vi "n3_bis_betas.vi"(4 "Time":dbl[](array[numeric]), 5 "Tamaño Sn":i32[](array[numeric]), 6 "Analysis":u8, 8 "m":dbl, 9 "P":dbl, 10 "Segmentation A":dbl[](array[numeric]), 11 "Segmentation B":dbl[](array[numeric])) -> (0 "bB":dbl, 1 "X2_tau":dbl[][](array[numeric]), 2 "X2_i":dbl[][](array[numeric]), 3 "bA":dbl)   [LabVIEW 2015]
uses:
  <vilib>/Analysis/baseanly.llb/Mean (DBL).vi
  <vilib>/Analysis/NI_AALBase.lvlib
  <vilib>/Analysis/NI_AALPro.lvlib
panel:
  out "bB_anterior":dbl
  out "bA_anterior":dbl
  out "amplitude 2":dbl
  out "offset 2":dbl
  out "offset":dbl
  out "time":dbl[](array[numeric])
  out "amplitude":dbl
  out "output array 4":dbl[](array[numeric])
  out "Canelos":dbl[](array[numeric])
  out "MA 3":dbl
  out "MB 2":dbl
  out "MA 2":dbl
  out "output array 2":dbl[](array[numeric])
  out "MB":dbl
  out "MA":dbl
  out "output array":dbl[](array[numeric])
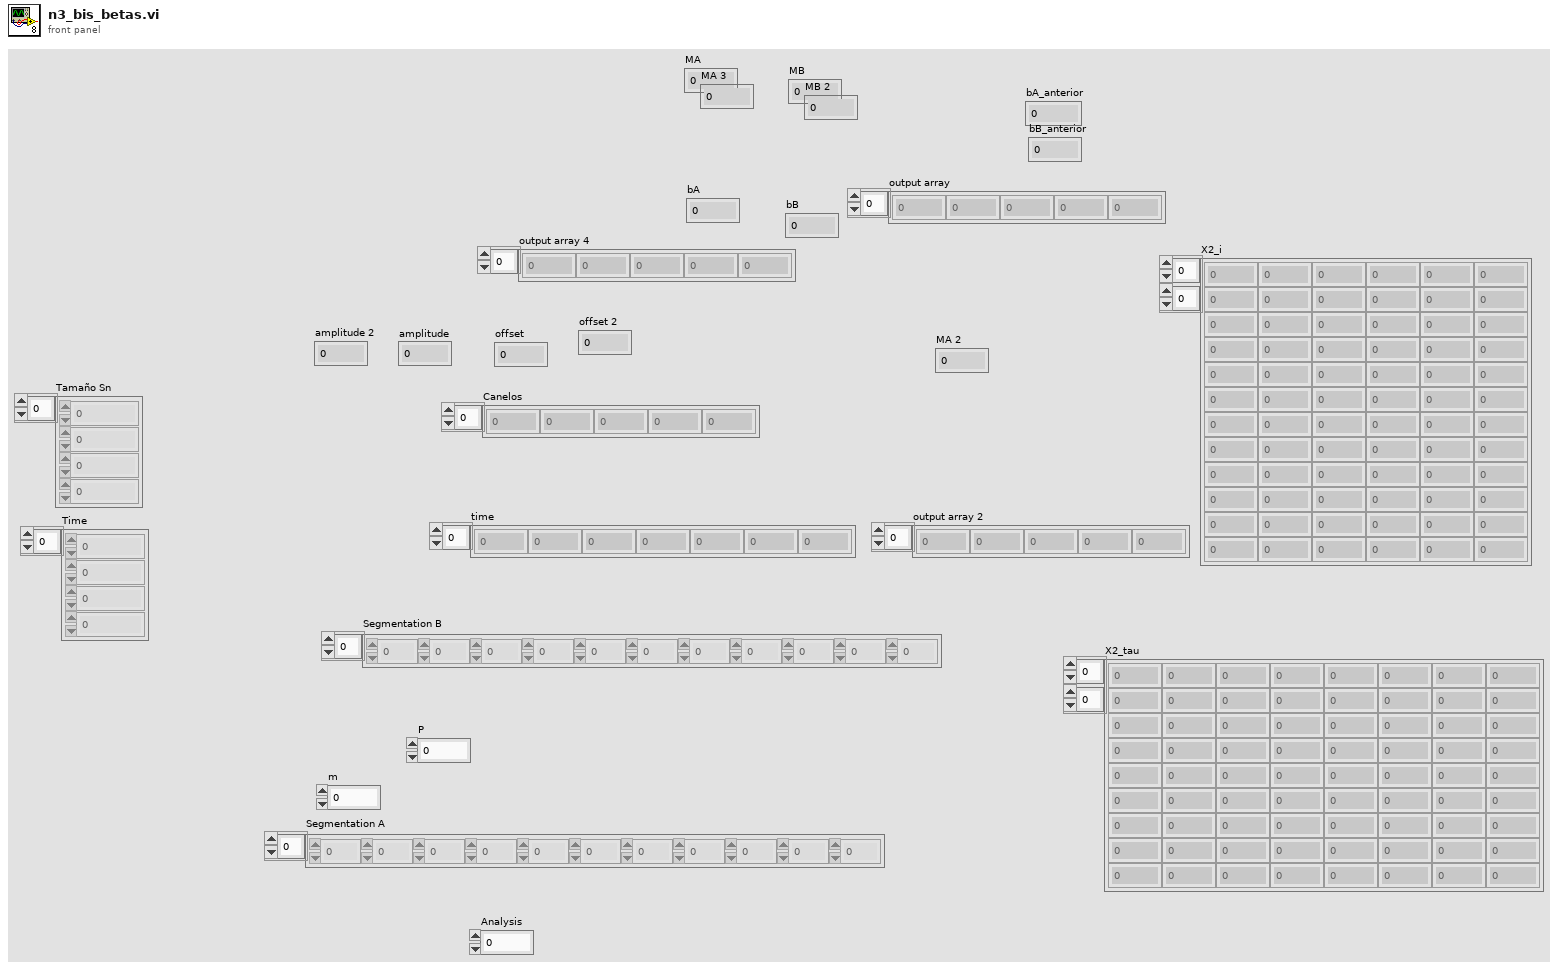
[diagram p1: front panel]
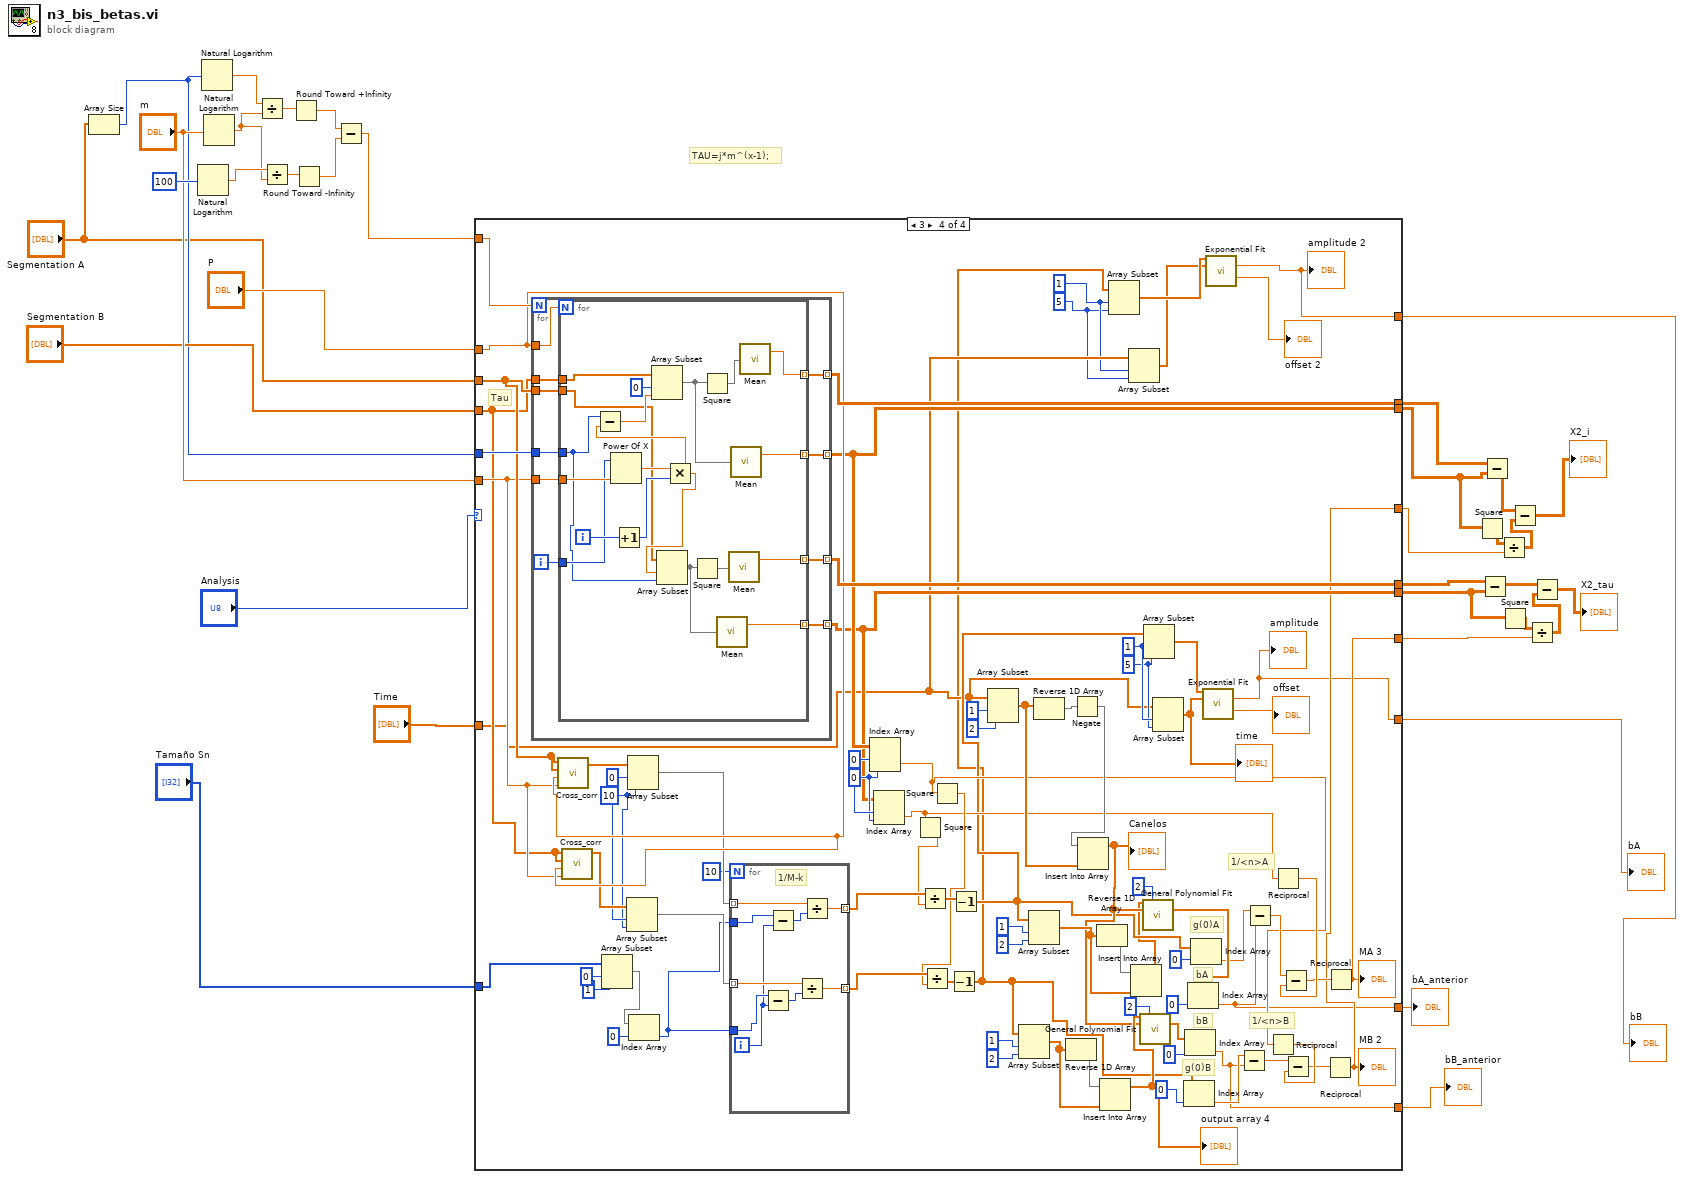
[diagram p0: block diagram]
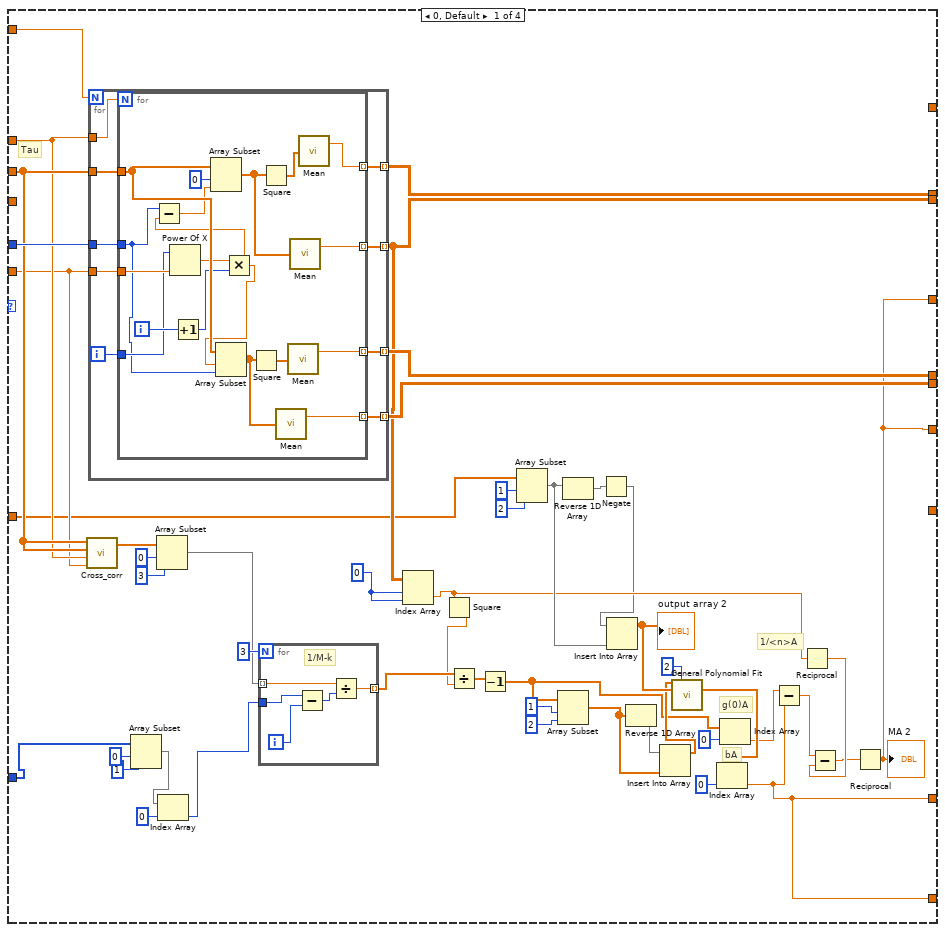
[diagram p2: hidden frame]
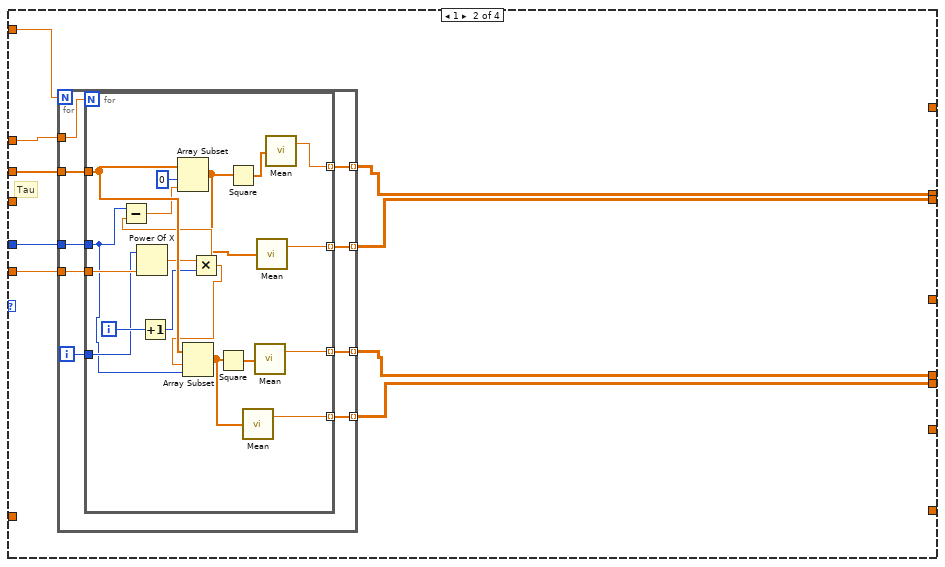
[diagram p3: hidden frame]
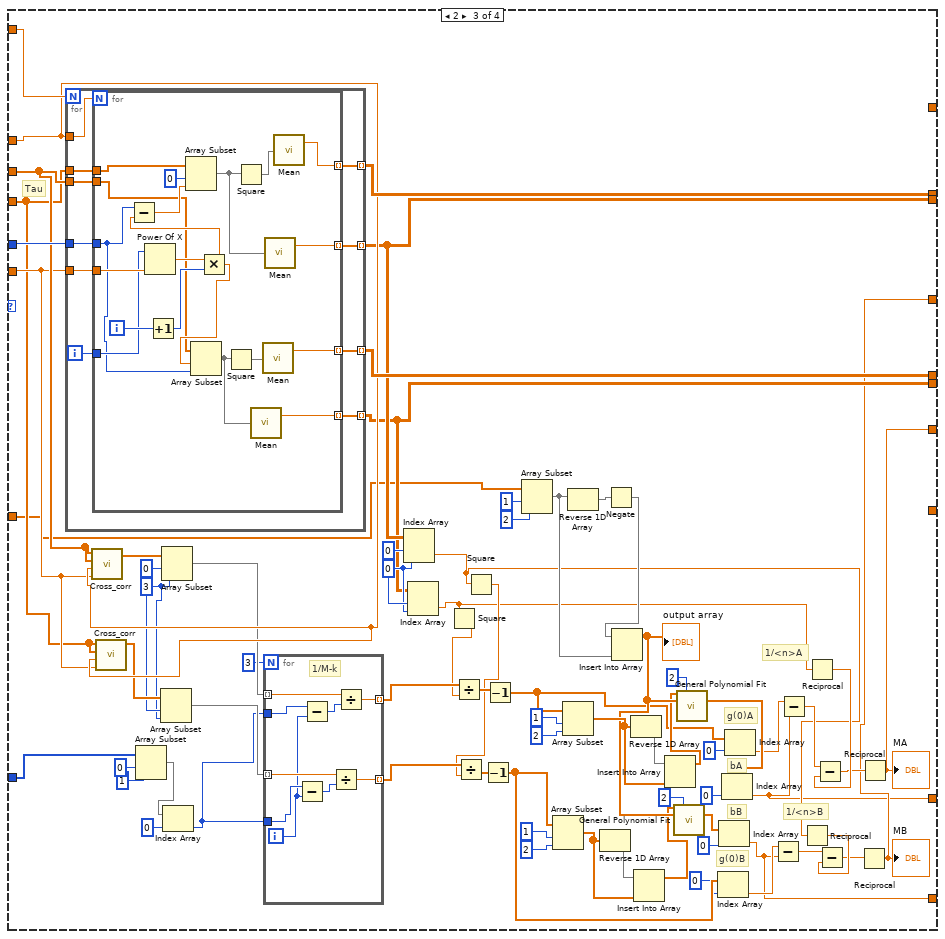
[diagram p4: hidden frame]
diagram:
  # "TAU=j*m^(x-1);"
  n1 = Array Size(array="Segmentation A") -> (size(s)=w20:i32)
  n2 = Natural Logarithm(1:100) -> (0:w32:dbl)
  n3 = Natural Logarithm(1:w20) -> (0:w35:dbl)
  n4 = Natural Logarithm(1:"m") -> (0:w31:dbl)
  n5 = Divide(x=w35, y=w31) -> (x/y=w34:dbl)
  n6 = Divide(x=w32, y=w31) -> (x/y=w29:dbl)
  n7 = Round Toward +Infinity(x=w34) -> (ceil(x): smallest int >= x=w30:dbl)
  n8 = Round Toward -Infinity(1:w29) -> (0:w28:dbl)
  n9 = Subtract(x=w30, y=w28) -> (x-y=w27:dbl)
  n10 = case shown="3" "Analysis" {
    tunnel: "Segmentation A" -> [w47 w124 w219 w341]
    tunnel: w20 -> [w79 w123 w222 w344]
    tunnel: w27 -> [w80 w122 w223 w345]
    tunnel: "m" -> [w45 w121 w217 w339]
    tunnel: "P" -> [w46 w120 w218 w340]
    tunnel: [w83 w119 w221 w343] -> w22
    tunnel: [w42 w118 w204 w326] -> w16
    tunnel: [w82 w117 w220 w342] -> w21
    tunnel: [w81 w116 w179 w304] -> w17
    tunnel: "Segmentation B" -> [_ _ w158 w285]
    tunnel: "Tamaño Sn" -> [w48 _ w210 w332]
    tunnel: [w41 _ w157 w284] -> w14
    tunnel: [w41 _ w156 w283] -> w9
    tunnel: "Time" -> [w37 _ w154 w270]
    tunnel: [w36 _ w153 w281] -> w2
    tunnel: [w36 _ w152 w280] -> w1
    tunnel: [_ _ _ w265] -> w4
    tunnel: [_ _ _ w264] -> w3
    frame 0, Default {
      w43 = 0 ("index (col)")
      # "1/<n>A"
      # "bA"
      # "g(0)A"
      # "Tau"
      n11 = call "Cross_corr.vi"("m"=w45, "P"=w46, "input B"=w47, "input A"=w47) -> ("Acc"=w78:dbl[])  [unwired: 5 in, 2 out]
      n12 = for {
        N: w80 -> [_]
        tunnel: w46 -> [w97]
        tunnel: w47 -> [w96]
        tunnel: w79 -> [w95]
        tunnel: w45 -> [w94]
        tunnel: [w93] -> w83 mode=indexing
        tunnel: [w92] -> w42 mode=indexing
        tunnel: [w90] -> w82 mode=indexing
        tunnel: [w89] -> w81 mode=indexing
        i -> [w91]
        n13 = for {
          N: w97 -> [_]
          tunnel: w96 -> [w112]
          tunnel: w95 -> [w104]
          tunnel: w94 -> [w115]
          tunnel: w91 -> [w106]
          tunnel: [w114] -> w93 mode=indexing
          tunnel: [w113] -> w92 mode=indexing
          tunnel: [w110] -> w90 mode=indexing
          tunnel: [w109] -> w89 mode=indexing
          i -> [w108]
          n14 = Power Of X(1:w115, 2:w106) -> (0:w98:dbl)
          n15 = Increment(x=w108) -> (x+1=w107:i32)
          n16 = Multiply(x=w98, y=w107) -> (x*y=w105:dbl)
          n17 = Subtract(x=w104, y=w105) -> (x-y=w102:dbl)
          n18 = Array Subset(array=w112, index=0, length=w102) -> (w103:dbl[])
          n19 = Array Subset(array=w112, index=w105, length=w104) -> (w99:dbl[])
          n20 = Square(x=w99) -> (x^2=w111:dbl[])
          n21 = Square(x=w103) -> (x^2=w100:dbl[])
          n22 = call-poly <vilib>:"Mean.vi"("X"=w99) -> ("mean"=w109:dbl)  [unwired: 1 out]
          n23 = call-poly <vilib>:"Mean.vi"("X"=w111) -> ("mean"=w110:dbl)  [unwired: 1 out]
          n24 = call-poly <vilib>:"Mean.vi"("X"=w103) -> ("mean"=w113:dbl)  [unwired: 1 out]
          n25 = call-poly <vilib>:"Mean.vi"("X"=w100) -> ("mean"=w114:dbl)  [unwired: 1 out]
        }
      }
      n26 = Array Subset(array=w48, index=0, length=1) -> (w73:i32[])
      n27 = Array Subset(array=w78, index=0, length=3) -> (w39:dbl[])
      n28 = Index Array(array=w73, index=0) -> (element=w44:i32)
      n29 = for {
        N: 3 -> [_]
        tunnel: w39 -> [w87] mode=indexing
        tunnel: w44 -> [w86]
        tunnel: [w84] -> w71 mode=indexing
        i -> [w85]
        # "1/M-k"
        n30 = Subtract(x=w86, y=w85) -> (x-y=w88:i32)
        n31 = Divide(x=w87, y=w88) -> (x/y=w84:dbl)
      }
      n32 = Index Array(array=w42, index (row)=w43, index (col)=w43) -> (element=w52:dbl)
      n33 = Square(x=w52) -> (x^2=w58:dbl)
      n34 = Divide(x=w71, y=w58) -> (x/y=w70:dbl[])
      n35 = Decrement(x=w70) -> (x-1=w57:dbl[])
      n36 = Array Subset(array=w37, index=1, length=2) -> (w62:dbl[])
      n37 = Array Subset(array=w57, index=1, length=2) -> (w61:dbl[])
      n38 = Reverse 1D Array(array=w62) -> (reversed array=w67:dbl[])
      n39 = Negate(x=w67) -> (-x=w38:dbl[])
      n40 = Insert Into Array(array=w38, new element=w62) -> (w60:dbl[])  [unwired: 1 in]
      "output array 2" <- w60
      n41 = Reverse 1D Array(array=w61) -> (reversed array=w63:dbl[])
      n42 = Insert Into Array(array=w63, new element=w61) -> (w59:dbl[])  [unwired: 1 in]
      n43 = call <vilib>:"General Polynomial Fit.vi"("Y"=w59, "polynomial order"=2, "X"=w60) -> ("Polynomial Coefficients"=w55:dbl[])  [unwired: 9 in, 3 out]
      n44 = Index Array(array=w55, index=0) -> (element=w36:dbl)
      n45 = Index Array(array=w57, index=0) -> (element=w53:dbl)
      n46 = Subtract(x=w53, y=w36) -> (x-y=w51:dbl)
      n47 = Reciprocal(x=w52) -> (1/x=w50:dbl)
      n48 = Subtract(x=w51, y=w50) -> (x-y=w49:dbl)
      n49 = Reciprocal(x=w49) -> (1/x=w41:dbl)
      "MA 2" <- w41
    }
    frame 1 {
      # "Tau"
      n50 = for {
        N: w122 -> [_]
        tunnel: w120 -> [w133]
        tunnel: w124 -> [w132]
        tunnel: w123 -> [w131]
        tunnel: w121 -> [w130]
        tunnel: [w129] -> w119 mode=indexing
        tunnel: [w128] -> w118 mode=indexing
        tunnel: [w126] -> w117 mode=indexing
        tunnel: [w125] -> w116 mode=indexing
        i -> [w127]
        n51 = for {
          N: w133 -> [_]
          tunnel: w132 -> [w148]
          tunnel: w131 -> [w138]
          tunnel: w130 -> [w151]
          tunnel: w127 -> [w141]
          tunnel: [w150] -> w129 mode=indexing
          tunnel: [w149] -> w128 mode=indexing
          tunnel: [w146] -> w126 mode=indexing
          tunnel: [w144] -> w125 mode=indexing
          i -> [w143]
          n52 = Power Of X(1:w151, 2:w141) -> (0:w140:dbl)
          n53 = Increment(x=w143) -> (x+1=w142:i32)
          n54 = Multiply(x=w140, y=w142) -> (x*y=w139:dbl)
          n55 = Subtract(x=w138, y=w139) -> (x-y=w136:dbl)
          n56 = Array Subset(array=w148, index=0, length=w136) -> (w137:dbl[])
          n57 = Array Subset(array=w148, index=w139, length=w138) -> (w145:dbl[])
          n58 = Square(x=w145) -> (x^2=w147:dbl[])
          n59 = Square(x=w137) -> (x^2=w134:dbl[])
          n60 = call-poly <vilib>:"Mean.vi"("X"=w145) -> ("mean"=w144:dbl)  [unwired: 1 out]
          n61 = call-poly <vilib>:"Mean.vi"("X"=w147) -> ("mean"=w146:dbl)  [unwired: 1 out]
          n62 = call-poly <vilib>:"Mean.vi"("X"=w137) -> ("mean"=w149:dbl)  [unwired: 1 out]
          n63 = call-poly <vilib>:"Mean.vi"("X"=w134) -> ("mean"=w150:dbl)  [unwired: 1 out]
        }
      }
    }
    frame 2 {
      w202 = 0 ("index (col)")
      w203 = 0 ("index (row)")
      w155 = 3 ("length")
      w214 = 0 ("index")
      # "1/<n>B"
      # "1/<n>A"
      # "bB"
      # "bA"
      # "g(0)B"
      # "g(0)A"
      # "Tau"
      n64 = for {
        N: w223 -> [_]
        tunnel: w218 -> [w242]
        tunnel: w158 -> [w241]
        tunnel: w222 -> [w240]
        tunnel: w217 -> [w239]
        tunnel: [w238] -> w221 mode=indexing
        tunnel: [w237] -> w204 mode=indexing
        tunnel: [w235] -> w220 mode=indexing
        tunnel: [w234] -> w179 mode=indexing
        tunnel: w219 -> [w233]
        i -> [w236]
        n65 = for {
          N: w242 -> [_]
          tunnel: w241 -> [w244]
          tunnel: w240 -> [w249]
          tunnel: w239 -> [w261]
          tunnel: w236 -> [w252]
          tunnel: [w260] -> w238 mode=indexing
          tunnel: [w259] -> w237 mode=indexing
          tunnel: [w257] -> w235 mode=indexing
          tunnel: [w255] -> w234 mode=indexing
          tunnel: w233 -> [w243]
          i -> [w254]
          n66 = Power Of X(1:w261, 2:w252) -> (0:w251:dbl)
          n67 = Increment(x=w254) -> (x+1=w253:i32)
          n68 = Multiply(x=w251, y=w253) -> (x*y=w250:dbl)
          n69 = Subtract(x=w249, y=w250) -> (x-y=w247:dbl)
          n70 = Array Subset(array=w244, index=0, length=w247) -> (w248:dbl[])
          n71 = Array Subset(array=w243, index=w250, length=w249) -> (w256:dbl[])
          n72 = Square(x=w256) -> (x^2=w258:dbl[])
          n73 = Square(x=w248) -> (x^2=w245:dbl[])
          n74 = call-poly <vilib>:"Mean.vi"("X"=w256) -> ("mean"=w255:dbl)  [unwired: 1 out]
          n75 = call-poly <vilib>:"Mean.vi"("X"=w258) -> ("mean"=w257:dbl)  [unwired: 1 out]
          n76 = call-poly <vilib>:"Mean.vi"("X"=w248) -> ("mean"=w259:dbl)  [unwired: 1 out]
          n77 = call-poly <vilib>:"Mean.vi"("X"=w245) -> ("mean"=w260:dbl)  [unwired: 1 out]
        }
      }
      n78 = call "Cross_corr.vi"("m"=w217, "P"=w218, "input B"=w219, "input A"=w219) -> ("Acc"=w216:dbl[])  [unwired: 5 in, 2 out]
      n79 = call "Cross_corr.vi"("m"=w217, "P"=w218, "input B"=w158, "input A"=w158) -> ("Acc"=w215:dbl[])  [unwired: 5 in, 2 out]
      n80 = Array Subset(array=w210, index=0, length=1) -> (w207:i32[])
      n81 = Array Subset(array=w215, index=w214, length=w155) -> (w212:dbl[])
      n82 = Array Subset(array=w216, index=w214, length=w155) -> (w213:dbl[])
      n83 = Index Array(array=w207, index=0) -> (element=w205:i32)
      n84 = for {
        N: 3 -> [_]
        tunnel: [w232] -> w200 mode=indexing
        tunnel: w212 -> [w231] mode=indexing
        tunnel: w205 -> [w229]
        tunnel: w213 -> [w227] mode=indexing
        tunnel: w205 -> [w226]
        tunnel: [w224] -> w201 mode=indexing
        i -> [w225]
        # "1/M-k"
        n85 = Subtract(x=w229, y=w225) -> (x-y=w230:i32)
        n86 = Subtract(x=w226, y=w225) -> (x-y=w228:i32)
        n87 = Divide(x=w231, y=w230) -> (x/y=w232:dbl)
        n88 = Divide(x=w227, y=w228) -> (x/y=w224:dbl)
      }
      n89 = Index Array(array=w204, index (row)=w203, index (col)=w202) -> (element=w160:dbl)
      n90 = Index Array(array=w179, index (row)=w203, index (col)=w202) -> (element=w167:dbl)
      n91 = Square(x=w167) -> (x^2=w177:dbl)
      n92 = Divide(x=w201, y=w177) -> (x/y=w199:dbl[])
      n93 = Square(x=w160) -> (x^2=w178:dbl)
      n94 = Divide(x=w200, y=w178) -> (x/y=w198:dbl[])
      n95 = Decrement(x=w198) -> (x-1=w174:dbl[])
      n96 = Decrement(x=w199) -> (x-1=w176:dbl[])
      n97 = Array Subset(array=w154, index=1, length=2) -> (w189:dbl[])
      n98 = Array Subset(array=w174, index=1, length=2) -> (w183:dbl[])
      n99 = Array Subset(array=w176, index=1, length=2) -> (w188:dbl[])
      n100 = Reverse 1D Array(array=w189) -> (reversed array=w195:dbl[])
      n101 = Reverse 1D Array(array=w183) -> (reversed array=w184:dbl[])
      n102 = Negate(x=w195) -> (-x=w194:dbl[])
      n103 = Insert Into Array(array=w194, new element=w189) -> (w182:dbl[])  [unwired: 1 in]
      "output array" <- w182
      n104 = Reverse 1D Array(array=w188) -> (reversed array=w190:dbl[])
      n105 = Insert Into Array(array=w184, new element=w183) -> (w180:dbl[])  [unwired: 1 in]
      n106 = Insert Into Array(array=w190, new element=w188) -> (w181:dbl[])  [unwired: 1 in]
      n107 = call <vilib>:"General Polynomial Fit.vi"("Y"=w180, "polynomial order"=2, "X"=w182) -> ("Polynomial Coefficients"=w170:dbl[])  [unwired: 9 in, 3 out]
      n108 = call <vilib>:"General Polynomial Fit.vi"("Y"=w181, "polynomial order"=2, "X"=w182) -> ("Polynomial Coefficients"=w172:dbl[])  [unwired: 9 in, 3 out]
      n109 = Index Array(array=w174, index=0) -> (element=w159:dbl)
      n110 = Index Array(array=w170, index=0) -> (element=w152:dbl)
      n111 = Index Array(array=w172, index=0) -> (element=w153:dbl)
      n112 = Index Array(array=w176, index=0) -> (element=w168:dbl)
      n113 = Subtract(x=w159, y=w152) -> (x-y=w163:dbl)
      n114 = Subtract(x=w168, y=w153) -> (x-y=w166:dbl)
      n115 = Reciprocal(x=w160) -> (1/x=w164:dbl)
      n116 = Reciprocal(x=w167) -> (1/x=w165:dbl)
      n117 = Subtract(x=w166, y=w165) -> (x-y=w161:dbl)
      n118 = Subtract(x=w163, y=w164) -> (x-y=w162:dbl)
      n119 = Reciprocal(x=w162) -> (1/x=w156:dbl)
      "MB" <- w156
      n120 = Reciprocal(x=w161) -> (1/x=w157:dbl)
      "MA" <- w157
    }
    frame 3 {
      w268 = 5 ("length")
      w269 = 1 ("index")
      w275 = 5 ("length")
      w276 = 1 ("index")
      w324 = 0 ("index (col)")
      w325 = 0 ("index (row)")
      w282 = 10 ("length")
      w336 = 0 ("index")
      # "1/<n>B"
      # "1/<n>A"
      # "bB"
      # "bA"
      # "g(0)B"
      # "g(0)A"
      # "Tau"
      n121 = for {
        N: w345 -> [_]
        tunnel: w340 -> [w364]
        tunnel: w285 -> [w363]
        tunnel: w344 -> [w362]
        tunnel: w339 -> [w361]
        tunnel: [w360] -> w343 mode=indexing
        tunnel: [w359] -> w326 mode=indexing
        tunnel: [w357] -> w342 mode=indexing
        tunnel: [w356] -> w304 mode=indexing
        tunnel: w341 -> [w355]
        i -> [w358]
        n122 = for {
          N: w364 -> [_]
          tunnel: w363 -> [w366]
          tunnel: w362 -> [w371]
          tunnel: w361 -> [w383]
          tunnel: w358 -> [w374]
          tunnel: [w382] -> w360 mode=indexing
          tunnel: [w381] -> w359 mode=indexing
          tunnel: [w379] -> w357 mode=indexing
          tunnel: [w377] -> w356 mode=indexing
          tunnel: w355 -> [w365]
          i -> [w376]
          n123 = Power Of X(1:w383, 2:w374) -> (0:w373:dbl)
          n124 = Increment(x=w376) -> (x+1=w375:i32)
          n125 = Multiply(x=w373, y=w375) -> (x*y=w372:dbl)
          n126 = Subtract(x=w371, y=w372) -> (x-y=w369:dbl)
          n127 = Array Subset(array=w366, index=0, length=w369) -> (w370:dbl[])
          n128 = Array Subset(array=w365, index=w372, length=w371) -> (w378:dbl[])
          n129 = Square(x=w378) -> (x^2=w380:dbl[])
          n130 = Square(x=w370) -> (x^2=w367:dbl[])
          n131 = call-poly <vilib>:"Mean.vi"("X"=w378) -> ("mean"=w377:dbl)  [unwired: 1 out]
          n132 = call-poly <vilib>:"Mean.vi"("X"=w380) -> ("mean"=w379:dbl)  [unwired: 1 out]
          n133 = call-poly <vilib>:"Mean.vi"("X"=w370) -> ("mean"=w381:dbl)  [unwired: 1 out]
          n134 = call-poly <vilib>:"Mean.vi"("X"=w367) -> ("mean"=w382:dbl)  [unwired: 1 out]
        }
      }
      n135 = call "Cross_corr.vi"("m"=w339, "P"=w340, "input B"=w341, "input A"=w341) -> ("Acc"=w338:dbl[])  [unwired: 5 in, 2 out]
      n136 = call "Cross_corr.vi"("m"=w339, "P"=w340, "input B"=w285, "input A"=w285) -> ("Acc"=w337:dbl[])  [unwired: 5 in, 2 out]
      n137 = Array Subset(array=w332, index=0, length=1) -> (w329:i32[])
      n138 = Array Subset(array=w337, index=w336, length=w282) -> (w334:dbl[])
      n139 = Array Subset(array=w338, index=w336, length=w282) -> (w335:dbl[])
      n140 = Index Array(array=w329, index=0) -> (element=w327:i32)
      n141 = for {
        N: 10 -> [_]
        tunnel: [w354] -> w322 mode=indexing
        tunnel: w334 -> [w353] mode=indexing
        tunnel: w327 -> [w351]
        tunnel: w335 -> [w349] mode=indexing
        tunnel: w327 -> [w348]
        tunnel: [w346] -> w323 mode=indexing
        i -> [w347]
        # "1/M-k"
        n142 = Subtract(x=w351, y=w347) -> (x-y=w352:i32)
        n143 = Subtract(x=w348, y=w347) -> (x-y=w350:i32)
        n144 = Divide(x=w353, y=w352) -> (x/y=w354:dbl)
        n145 = Divide(x=w349, y=w350) -> (x/y=w346:dbl)
      }
      n146 = Index Array(array=w326, index (row)=w325, index (col)=w324) -> (element=w287:dbl)
      n147 = Index Array(array=w304, index (row)=w325, index (col)=w324) -> (element=w294:dbl)
      n148 = Square(x=w294) -> (x^2=w302:dbl)
      n149 = Divide(x=w323, y=w302) -> (x/y=w321:dbl[])
      n150 = Square(x=w287) -> (x^2=w303:dbl)
      n151 = Divide(x=w322, y=w303) -> (x/y=w320:dbl[])
      n152 = Decrement(x=w320) -> (x-1=w266:dbl[])
      n153 = Decrement(x=w321) -> (x-1=w273:dbl[])
      n154 = Array Subset(array=w270, index=1, length=2) -> (w311:dbl[])
      n155 = Array Subset(array=w266, index=1, length=2) -> (w305:dbl[])
      n156 = Array Subset(array=w273, index=1, length=2) -> (w310:dbl[])
      n157 = Reverse 1D Array(array=w311) -> (reversed array=w317:dbl[])
      n158 = Reverse 1D Array(array=w305) -> (reversed array=w306:dbl[])
      n159 = Negate(x=w317) -> (-x=w316:dbl[])
      n160 = Insert Into Array(array=w316, new element=w311) -> (w278:dbl[])  [unwired: 1 in]
      "Canelos" <- w278
      n161 = Reverse 1D Array(array=w310) -> (reversed array=w312:dbl[])
      n162 = Insert Into Array(array=w306, new element=w305) -> (w279:dbl[])  [unwired: 1 in]
      "output array 4" <- w279
      n163 = Array Subset(array=w266, index=w269, length=w268) -> (w263:dbl[])
      n164 = Array Subset(array=w270, index=w269, length=w268) -> (w262:dbl[])
      n165 = Insert Into Array(array=w312, new element=w310) -> (w271:dbl[])  [unwired: 1 in]
      n166 = call <vilib>:"General Polynomial Fit.vi"("Y"=w279, "polynomial order"=2, "X"=w278) -> ("Polynomial Coefficients"=w297:dbl[])  [unwired: 9 in, 3 out]
      n167 = call <vilib>:"General Polynomial Fit.vi"("Y"=w271, "polynomial order"=2, "X"=w278) -> ("Polynomial Coefficients"=w299:dbl[])  [unwired: 9 in, 3 out]
      n168 = Array Subset(array=w273, index=w276, length=w275) -> (w277:dbl[])
      n169 = Array Subset(array=w270, index=w276, length=w275) -> (w274:dbl[])
      "time" <- w274
      n170 = Index Array(array=w266, index=0) -> (element=w286:dbl)
      n171 = Index Array(array=w297, index=0) -> (element=w280:dbl)
      n172 = Index Array(array=w299, index=0) -> (element=w281:dbl)
      n173 = Index Array(array=w273, index=0) -> (element=w295:dbl)
      n174 = call <vilib>:"Exponential Fit.vi"("Y"=w277, "X"=w274) -> ("amplitude"=w264:dbl, "offset"=→"offset":dbl)  [unwired: 8 in, 4 out]
      "amplitude" <- w264
      n175 = call <vilib>:"Exponential Fit.vi"("Y"=w263, "X"=w262) -> ("amplitude"=w265:dbl, "offset"=→"offset 2":dbl)  [unwired: 8 in, 4 out]
      "amplitude 2" <- w265
      n176 = Subtract(x=w286, y=w280) -> (x-y=w290:dbl)
      n177 = Subtract(x=w295, y=w281) -> (x-y=w293:dbl)
      n178 = Reciprocal(x=w287) -> (1/x=w291:dbl)
      n179 = Reciprocal(x=w294) -> (1/x=w292:dbl)
      n180 = Subtract(x=w293, y=w292) -> (x-y=w288:dbl)
      n181 = Subtract(x=w290, y=w291) -> (x-y=w289:dbl)
      n182 = Reciprocal(x=w289) -> (1/x=w283:dbl)
      "MB 2" <- w283
      n183 = Reciprocal(x=w288) -> (1/x=w284:dbl)
      "MA 3" <- w284
    }
  }
  "bA" <- w3
  "bB" <- w4
  "bA_anterior" <- w2
  "bB_anterior" <- w1
  n184 = Square(x=w16) -> (x^2=w8:dbl[][])
  n185 = Subtract(x=w21, y=w17) -> (x-y=w11:dbl[][])
  n186 = Subtract(x=w22, y=w16) -> (x-y=w15:dbl[][])
  n187 = Divide(x=w8, y=w9) -> (x/y=w7:dbl[][])
  n188 = Square(x=w17) -> (x^2=w13:dbl[][])
  n189 = Subtract(x=w15, y=w7) -> (x-y=→"X2_i":dbl[][])
  n190 = Divide(x=w13, y=w14) -> (x/y=w12:dbl[][])
  n191 = Subtract(x=w11, y=w12) -> (x-y=→"X2_tau":dbl[][])
